vi "CPCconcentration.vi"() -> ()   [LabVIEW 2011, in "CPCconc.lvlib"]
uses:
  CPCconc.lvlib
panel:
  in  "CPCconc":dbl
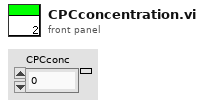
[diagram p1: front panel]
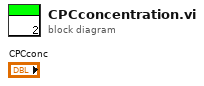
[diagram p0: block diagram]
diagram:
